vi "Get Acq Raw Params.vi"(0 "raw display notifier":refnum<notifier>, 7 "Channel Configurations":refnum<vi>, 11 "error in (no error)":errorcluster) -> (15 "error out":errorcluster)   [LabVIEW 2023, in "GettingStarted_Acq_148X_Host.lvlib"]
uses:
  GettingStarted_Acq_148X_Host.lvlib
  Common/Types/Serial Channel Display Parameters.ctl
  <vilib>/vision/Image Controls.llb/IMAQ Image.ctl
  Common/Types/RAW Interpretation for Display.ctl
  <instrlib>/FlexRIO/Automotive Vision Utility/v1/Host/Automotive Vision Utility.lvlib
  Common/GettingStarted_Common_148X_Host.lvlib
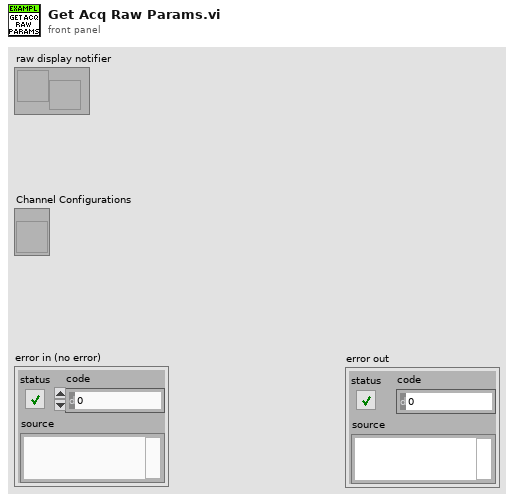
[diagram p1: front panel]
types:
  T1 = typedef "GettingStarted_Common_148X_Host.lvlib/Serial Channel Display Parameters.ctl" = cluster{"images":cluster{"grayscale":T2, "color":T2}, "RAW parameters":cluster{"interpretation":T3, "bayer parameters":cluster{"pattern":i32, "algorithm":i32, "red gain":dbl, "green gain":dbl, "blue gain":dbl}}}
  T2 = typedef "IMAQ Image.ctl" = refnum<image>
  T3 = typedef "GettingStarted_Common_148X_Host.lvlib/RAW Interpretation for Display.ctl" = enum16{"Grayscale", "Bayer", "RGB", "YUV422", "YUV420", "Legacy YUV420"}
  T4 = typedef "GettingStarted_Common_148X_Host.lvlib/Serial Channel Configuration.ctl" = cluster{"Serial Channel":string, "FPGA Display Parameters":T5, "RAW Display Parameters":cluster{"Interpretation":T3, "Bayer Parameters":cluster{"Pattern":i32, "Algorithm":i32, "Red Gain":dbl, "Green Gain":dbl, "Blue Gain":dbl}}}
  T5 = typedef "NI CSI-2 API FPGA v2.lvlib/Display Parameters.ctl" = cluster{"virtual channel":fxp<+,4,4>, "payload data type":T6, "frame skip count":u16, "line skip count":u8, "pixel skip count":fxp<+,5,5>}
  T6 = typedef "NI CSI-2 API Common v2.lvlib/LLP Data Type.ctl" = enum8{"Frame Start", "Frame End", "Line Start", "Line End", "End of Transmission", "Reserved 0", "Reserved 1", "Reserved 2", "Generic Short Packet 1", "Generic Short Packet 2", "Generic Short Packet 3", "Generic Short Packet 4", "Generic Short Packet 5", "Generic Short Packet 6", "Generic Short Packet 7", "Generic Short Packet 8", "Null", "Blanking Data", "Embedded 8-bit non Image Data", "Generic Long Packet 1", "Generic Long Packet 2", "Generic Long Packet 3", "Generic Long Packet 4", "Reserved 3", "YUV420 8-bit", "YUV420 10-bit", "Legacy YUV420 8-bit", "Reserved 4", "YUV420 8-bit Chroma Shifted", "YUV420 10-bit Chroma Shifted", "YUV422 8-bit", "YUV422 10-bit", "RGB444", "RGB555", "RGB565", "RGB666", "RGB888", "Reserved 5", "Reserved 6", "RAW 24", "RAW 6", "RAW 7", "RAW 8", "RAW 10", "RAW 12", "RAW 14", "RAW 16", "RAW 20", "User Defined 8-bit Data 1", "User Defined 8-bit Data 2", "User Defined 8-bit Data 3", "User Defined 8-bit Data 4", "User Defined 8-bit Data 5", "User Defined 8-bit Data 6", "User Defined 8-bit Data 7", "User Defined 8-bit Data 8", "USL Command", "Reserved 7", "Reserved 8", "Reserved 9", "Reserved 10", "Reserved 11", "Reserved 12", "LRTE EPD Spacer"}
  T7 = cluster{"Interpretation":T3, "Bayer Parameters":cluster{"Pattern":i32, "Algorithm":i32, "Red Gain":dbl, "Green Gain":dbl, "Blue Gain":dbl}}
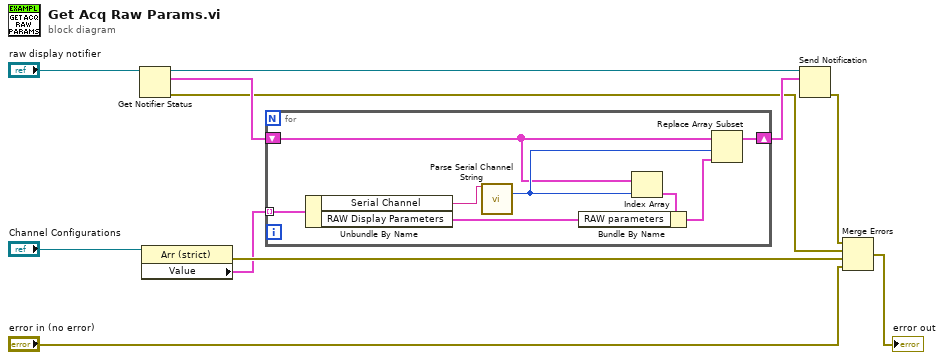
[diagram p0: block diagram]
diagram:
  n1 = Get Notifier Status(notifier="raw display notifier") -> (notifier out=w6:refnum<notifier>, current notification=w8:T1[], error out=w4:errorcluster)  [unwired: 1 in, 2 out]
  n2 = property class="Arr (strict)"(reference="Channel Configurations") -> (error out=w10:errorcluster, "Value"=w9:T4[])  [unwired: 1 in, 1 out]
  n3 = for {
    tunnel: w9 -> [w19] mode=indexing
    shift-right: [w12] -> w7
    shift-left: w8 -> [w14]
    n4 = Unbundle By Name(w19) -> ("Serial Channel"=w18:string, "RAW Display Parameters"=w15:T7)
    n5 = call <instrlib>:"Parse Serial Channel String.vi"("serial channel string"=w18) -> ("channel number"=w17:i32)  [unwired: 13 in, 1 out]
    n6 = Index Array(array=w14, index=w17) -> (element=w16:T1)
    n7 = Bundle By Name(cluster=w16, "RAW parameters"=w15) -> (w13:T1)
    n8 = Replace Array Subset(array=w14, new element=w13, index=w17) -> (w12:T1[])
  }
  n9 = Send Notification(notification=w7, notifier=w6) -> (error out=w5:errorcluster)  [unwired: 1 in, 1 out]
  n10 = Merge Errors(w5, w4, w10, "error in (no error)") -> (→"error out":errorcluster)
